vi "实时小时数据单参数上传.vi"() -> (4 "数据发送起始时间":timestamp format="%<%.3X\n%Y/%m/%d>T", 15 "error out":errorcluster)   [LabVIEW 2016, in "数据传输系统.lvlib"]
uses:
  <vilib>/Utility/config.llb/Write Key (String).vi
  <vilib>/Utility/config.llb/NI_LVConfig.lvlib
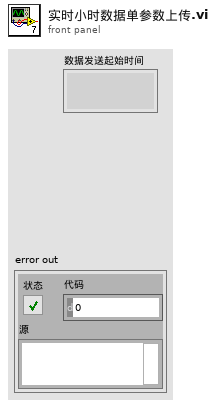
[diagram p1: front panel]
types:
  T1 = cluster{"CODMn":string, "CODCr":string, "DO":string, "铜":string, "PH":string, "氨氮":string, "比电导率":string, "水温":string, "COD":string, "浊度":string, "总氮":string, "总磷":string, "叶绿素a":string, "藻密度":string, "水位":string, "流速":string, "瞬时流量":string, "累积流量":string, "亚硝酸盐":string, "硫化物":string, "ORP":string, "铅":string, "镉":string, "锌":string, "镍":string, "锰":string, "汞":string, "气温":string, "气压":string, "风速":string, "风向":string}
  T2 = cluster{"setini":string, "sysini":string, "hechaini":string, "actualwrite":string, "actualread":string, "datasent":string, "反控命令信息队列":string, "反控与仪器交互":string}
  T3 = cluster{"time1":string, "time2":string, "time3":string, "time4":string, "time5":string, "time6":string, "time7":string, "time8":string, "time9":string, "time10":string, "time11":string, "time12":string, "time13":string, "time14":string, "time15":string, "time16":string, "time17":string, "time18":string, "time19":string, "time20":string, "time21":string, "time22":string, "time23":string, "time24":string, "time25":string, "time26":string, "time27":string, "time28":string, "time29":string, "time30":string, "time31":string}
  T4 = typedef "NI_LVConfig.lvlib/Config Data RefNum.ctl" = refnum<k1>
  T5 = cluster{"水样数据索引[0]":string, "水样数据索引[1]":string, "水样数据索引[2]":string, "水样数据索引[3]":string, "水样数据索引[4]":string, "水样数据索引[5]":string, "水样数据索引[6]":string, "水样数据索引[7]":string, "水样数据索引[8]":string, "水样数据索引[9]":string, "水样数据索引[10]":string, "水样数据索引[11]":string, "水样数据索引[12]":string, "水样数据索引[13]":string, "水样数据索引[14]":string, "水样数据索引[15]":string, "水样数据索引[16]":string, "水样数据索引[17]":string, "水样数据索引[18]":string, "水样数据索引[19]":string, "水样数据索引[20]":string, "水样数据索引[21]":string, "水样数据索引[22]":string, "水样数据索引[23]":string, "水样数据索引[24]":string, "水样数据索引[25]":string, "水样数据索引[26]":string, "水样数据索引[27]":string, "水样数据索引[28]":string, "水样数据索引[29]":string, "水样数据索引[30]":string}
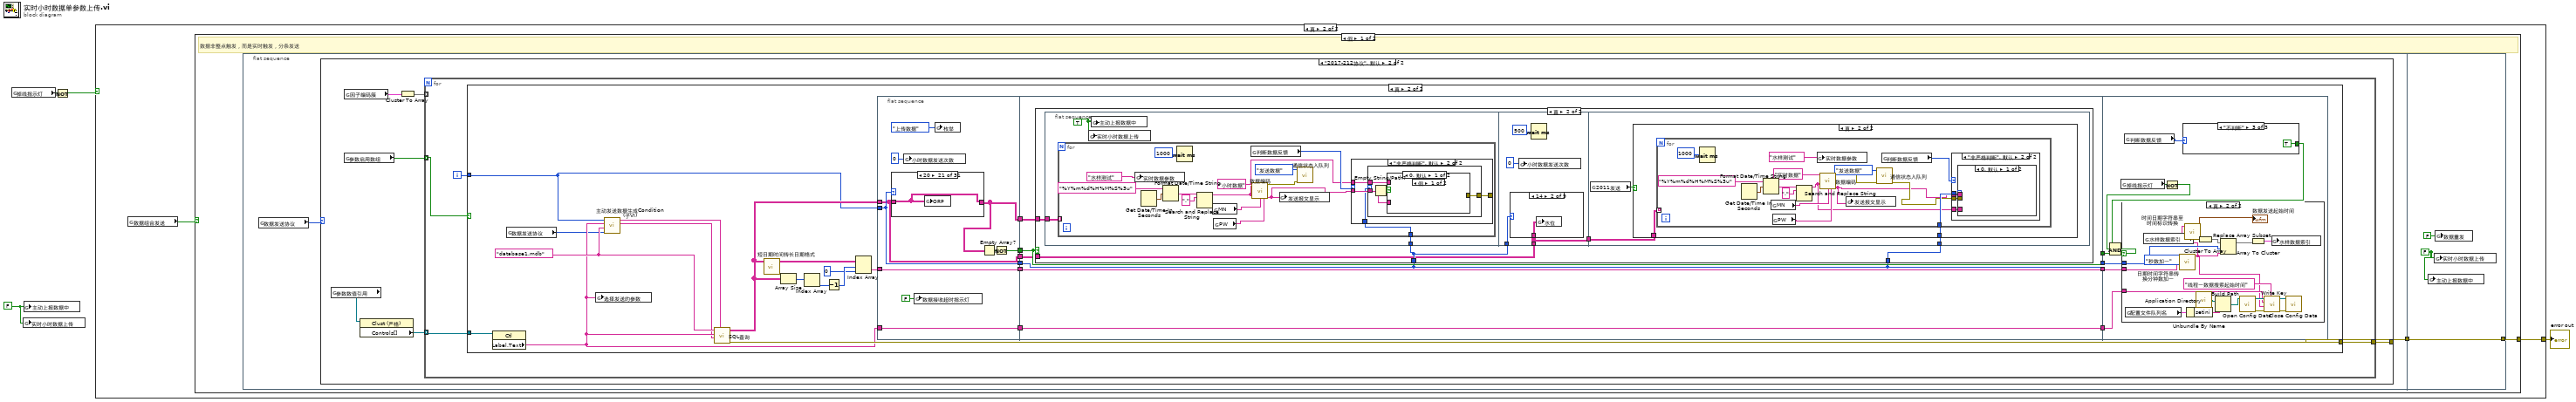
[diagram p0: block diagram]
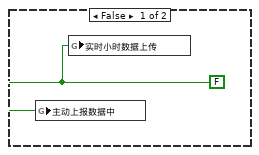
[diagram p2: hidden frame]
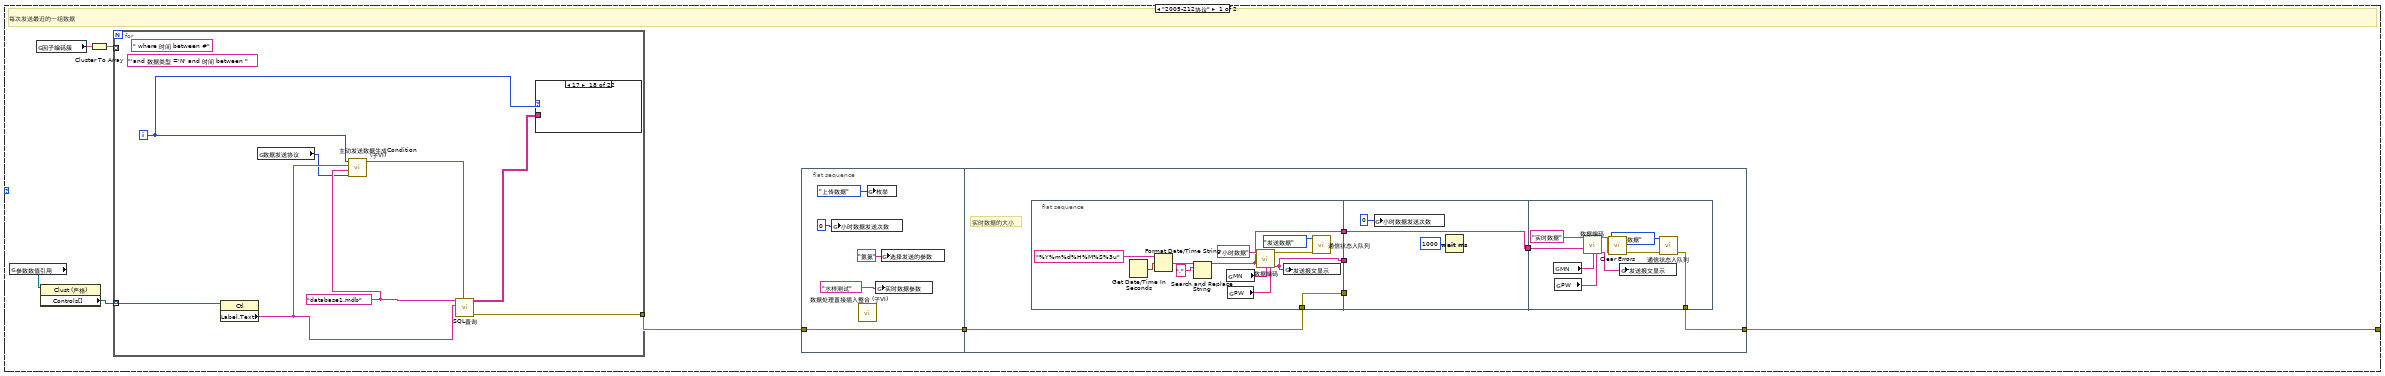
[diagram p3: hidden frame]
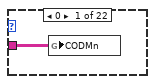
[diagram p4: hidden frame]
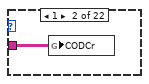
[diagram p5: hidden frame]
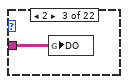
[diagram p6: hidden frame]
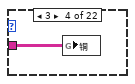
[diagram p7: hidden frame]
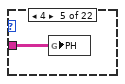
[diagram p8: hidden frame]
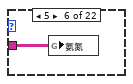
[diagram p9: hidden frame]
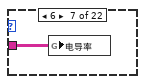
[diagram p10: hidden frame]
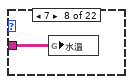
[diagram p11: hidden frame]
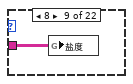
[diagram p12: hidden frame]
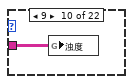
[diagram p13: hidden frame]
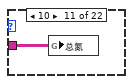
[diagram p14: hidden frame]
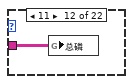
[diagram p15: hidden frame]
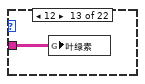
[diagram p16: hidden frame]
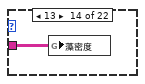
[diagram p17: hidden frame]
diagram:
  w1 = FALSE ("小时数据上传")
  n1 = global read "全局 数据发送重叠.vi" "掉线指示灯"() -> (w4:bool)
  n2 = global write "全局1.vi" "实时小时数据上传"(w1) -> ()
  n3 = global write "全局 数据发送重叠.vi" "主动上报数据中"(w1) -> ()
  n4 = Not(x=w4) -> (.not. x?=w3:bool)
  n5 = case shown="真" w3 {
    tunnel: [_ w7] -> w2
    frame False {
      w5 = FALSE ("小时数据上传")
      n6 = global write "全局 数据发送重叠.vi" "主动上报数据中"(w5) -> ()
      n7 = global write "全局1.vi" "实时小时数据上传"(w5) -> ()
    }
    frame True {
      n8 = global read "断电保存全局.vi" "数据组合发送"() -> (w6:bool)
      n9 = case shown="假" w6 {
        tunnel: [w8 _] -> w7
        frame False {
          # "数据非整点触发，而是实时触发，分条发送"
          n10 = flat-sequence {
            tunnel: [w11] -> w9
            tunnel: [w271] -> w8
            tunnel: w9 -> [w271]
            frame #0 {
              n11 = global read "断电保存全局.vi" "数据发送协议"() -> (w10:enum16{"2005-212协议", "2017-212协议"})
              n12 = case shown="\"2017-212协议\", 默认" w10 {
                tunnel: [w14 w83] -> w11
                frame "2005-212协议" {
                  # "每次发送最近的一组数据"
                  n13 = global read "断电保存全局.vi" "参数数值引用"() -> (w12:refnum<vi>)
                  n14 = global read "断电保存全局.vi" "因子编码簇"() -> (w13:T1)
                  n15 = property class="Clust (严格)"(reference=w12) -> ("Controls[]"=w15:refnum<vi>[])  [unwired: 1 in, 2 out]
                  n16 = Cluster To Array(cluster=w13) -> (array=w18:string[])
                  n17 = for {
                    tunnel: w18 -> [_] mode=indexing
                    tunnel: [w61] -> w17
                    tunnel: w15 -> [w56] mode=indexing
                    i -> [w54]
                    (unwired) " where 时间 between #"
                    w59 = "database1.mdb" ("database")
                    (unwired) "'and 数据类型 ='N' and 时间 between "
                    n18 = property class="Ctl"(reference=w56) -> ("Label.Text"=w60:string)  [unwired: 1 in, 2 out]
                    n19 = global read "断电保存全局.vi" "数据发送协议"() -> (w57:enum16{"2005-212协议", "2017-212协议"})
                    n20 = call "主动发送数据生成Condition(子VI).vi"("数据发送协议"=w57, "database"=w59, "Label.Text"=w60, "数值"=w54) -> ("CONDITION"=w58:string)  [unwired: 6 in, 1 out]
                    n21 = call "SQL查询.vi"("condition"=w58, "table输入"=w60, "database"=w59) -> ("error out"=w61:errorcluster, "data"=w55:string[][])  [unwired: 6 in, 1 out]
                    n22 = case shown="17" w54 {
                      tunnel: w55 -> [w62 w63 w64 w65 w66 w67 w68 w69 w70 w71 w72 w73 w74 w75 _ _ _ _ w76 w77 w78 _]
                      frame 0 {
                        n23 = global write "全局 所有参数.vi" "CODMn"(w62) -> ()
                      }
                      frame 1 {
                        n24 = global write "全局 所有参数.vi" "CODCr"(w63) -> ()
                      }
                      frame 2 {
                        n25 = global write "全局 所有参数.vi" "DO"(w64) -> ()
                      }
                      frame 3 {
                        n26 = global write "全局 所有参数.vi" "铜"(w65) -> ()
                      }
                      frame 4 {
                        n27 = global write "全局 所有参数.vi" "PH"(w66) -> ()
                      }
                      frame 5 {
                        n28 = global write "全局 所有参数.vi" "氨氮"(w67) -> ()
                      }
                      frame 6 {
                        n29 = global write "全局 所有参数.vi" "电导率"(w68) -> ()
                      }
                      frame 7 {
                        n30 = global write "全局 所有参数.vi" "水温"(w69) -> ()
                      }
                      frame 8 {
                        n31 = global write "全局 所有参数.vi" "盐度"(w70) -> ()
                      }
                      frame 9 {
                        n32 = global write "全局 所有参数.vi" "浊度"(w71) -> ()
                      }
                      frame 10 {
                        n33 = global write "全局 所有参数.vi" "总氮"(w72) -> ()
                      }
                      frame 11 {
                        n34 = global write "全局 所有参数.vi" "总磷"(w73) -> ()
                      }
                      frame 12 {
                        n35 = global write "全局 所有参数.vi" "叶绿素"(w74) -> ()
                      }
                      frame 13 {
                        n36 = global write "全局 所有参数.vi" "藻密度"(w75) -> ()
                      }
                      frame 14 {
                      }
                      frame 15 {
                      }
                      frame 16 {
                      }
                      frame 17 {
                      }
                      frame 18 {
                        n37 = global write "全局 所有参数.vi" "亚硝酸盐"(w76) -> ()
                      }
                      frame 19 {
                        n38 = global write "全局 所有参数.vi" "硫化物"(w77) -> ()
                      }
                      frame 20 {
                        n39 = global write "全局 所有参数.vi" "ORP"(w78) -> ()
                      }
                      frame 21, Default {
                      }
                    }
                  }
                  n40 = flat-sequence {
                    tunnel: w17 -> [w19]
                    tunnel: [w19] -> w16
                    tunnel: w16 -> [w27]
                    tunnel: [w26] -> w14
                    frame #0 {
                      n41 = global write "全局 小时数据发送次数.vi" "小时数据发送次数"(0 ("小时数据发送次数")) -> ()
                      n42 = call "数据处理直接插入整合 (子VI).vi"() -> ()  [unwired: 12 in]
                      n43 = global write "全局1.vi" "枚举"(enum16{"返回请求应答", "上传数据", "返回执行结果"}."上传数据" ("枚举")) -> ()
                      n44 = global write "全局 实时数据参数.vi" "实时数据参数"("水样测试" ("实时数据参数")) -> ()
                      n45 = global write "全局 水样时间.vi" "选择发送的参数"("氨氮" ("选择发送的参数")) -> ()
                    }
                    frame #1 {
                      # "实时数据的大小"
                      n46 = flat-sequence {
                        tunnel: [w36] -> w29
                        tunnel: [w31] -> w28
                        tunnel: w27 -> [w31]
                        tunnel: [w30] -> w25
                        tunnel: w29 -> [_]
                        tunnel: w28 -> [_]
                        tunnel: w25 -> [w42]
                        tunnel: [w42] -> w24
                        tunnel: [w47] -> w26
                        tunnel: w24 -> [w46]
                        frame #0 {
                          n47 = Get Date/Time In Seconds() -> (seconds since 1Jan1904=w39:timestamp)
                          n48 = Format Date/Time String(time format string (%c)="%Y%m%d%H%M%S%3u" ("时间格式字符串(%c)"), seconds (now)=w39) -> (date/time string=w40:string)  [unwired: 1 in]
                          n49 = Search and Replace String(input string=w40, search string="." ("搜索字符串")) -> (result string=w30:string)  [unwired: 6 in, 3 out]
                          n50 = global read "断电保存全局.vi" "MN"() -> (w34:string)
                          n51 = global read "断电保存全局.vi" "PW"() -> (w33:string)
                          n52 = call "数据编码.vi"("table输入"="小时数据" ("新元素/子数组"), "QN"=w30, "MN"=w34, "PW"=w33) -> ("错误常量"=w32:errorcluster, "通讯包字符串"=w36:string)  [unwired: 10 in]
                          n53 = global write "全局1.vi" "发送报文显示"(w36) -> ()
                          n54 = call "通信状态入队列.vi"("错误输入（无错误）"=w32, "枚举"=enum16{"打开连接", "发送数据", "读取数据", "数据处理", "关闭连接"}."发送数据") -> ()  [unwired: 9 in, 1 out]
                        }
                        frame #1 {
                          n55 = global write "全局 小时数据发送次数.vi" "小时数据发送次数"(0 ("小时数据发送次数")) -> ()
                          n56 = Wait (ms)(milliseconds to wait=u32 1000 ("等待时间（毫秒）")) -> ()  [unwired: 1 out]
                        }
                        frame #2 {
                          n57 = global read "断电保存全局.vi" "MN"() -> (w49:string)
                          n58 = global read "断电保存全局.vi" "PW"() -> (w50:string)
                          n59 = call "数据编码.vi"("table输入"="实时数据" ("新元素/子数组"), "QN"=w46, "MN"=w49, "PW"=w50) -> ("错误常量"=w48:errorcluster, "通讯包字符串"=w52:string)  [unwired: 10 in]
                          n60 = call <vilib>:"Clear Errors.vi"("error in (no error)"=w48) -> ("error out"=w45:errorcluster)  [unwired: 5 in, 1 out]
                          n61 = global write "全局1.vi" "发送报文显示"(w52) -> ()
                          n62 = call "通信状态入队列.vi"("错误输入（无错误）"=w45, "枚举"=enum16{"打开连接", "发送数据", "读取数据", "数据处理", "关闭连接"}."发送数据") -> ("错误输出"=w47:errorcluster)  [unwired: 9 in]
                        }
                      }
                    }
                  }
                }
                frame "2017-212协议", Default {
                  n63 = global read "断电保存全局.vi" "参数数值引用"() -> (w80:refnum<vi>)
                  n64 = global read "断电保存全局.vi" "参数启用数组"() -> (w79:bool[])
                  n65 = global read "断电保存全局.vi" "因子编码簇"() -> (w81:T1)
                  n66 = property class="Clust (严格)"(reference=w80) -> ("Controls[]"=w82:refnum<vi>[])  [unwired: 1 in, 2 out]
                  n67 = Cluster To Array(cluster=w81) -> (array=w84:string[])
                  n68 = for {
                    tunnel: w84 -> [_] mode=indexing
                    tunnel: [w88] -> w83
                    tunnel: w82 -> [w86] mode=indexing
                    tunnel: w79 -> [w85] mode=indexing
                    i -> [w87]
                    n69 = case shown="真" w85 {
                      tunnel: [_ w101] -> w88
                      tunnel: w87 -> [_ w92]
                      tunnel: w86 -> [_ w91]
                      frame False {
                      }
                      frame True {
                        w100 = "database1.mdb" ("database")
                        n70 = property class="Ctl"(reference=w91) -> ("Label.Text"=w99:string)  [unwired: 1 in, 2 out]
                        n71 = global read "断电保存全局.vi" "数据发送协议"() -> (w98:enum16{"2005-212协议", "2017-212协议"})
                        n72 = global write "全局 水样时间.vi" "选择发送的参数"(w99) -> ()
                        n73 = call "主动发送数据生成Condition(子VI).vi"("数据发送协议"=w98, "database"=w100, "Label.Text"=w99, "数值"=w92) -> ("columns"=w90:string[], "CONDITION"=w104:string)  [unwired: 6 in]
                        n74 = call "SQL查询.vi"("condition"=w104, "columns"=w90, "table输入"=w99, "database"=w100) -> ("error out"=w101:errorcluster, "data"=w95:string[][])  [unwired: 5 in, 1 out]
                        n75 = call "短日期时间转长日期格式.vi"("data"=w95) -> ("输出数组"=w103:string[][])  [unwired: 10 in]
                        n76 = Array Size(array=w95) -> (size(s)=w97:i32[])
                        n77 = Index Array(array=w97) -> (element=w96:i32)  [unwired: 1 in]
                        n78 = Decrement(x=w96) -> (x-1=w94:i32)
                        n79 = Index Array(array=w103, index (row)=w94, index (col)=0 ("禁用的索引 (列)")) -> (element=w102:string)
                        n80 = flat-sequence {
                          tunnel: [w115] -> w113
                          tunnel: [w116] -> w112
                          tunnel: w95 -> [w114]
                          tunnel: w92 -> [w119]
                          tunnel: w99 -> [w121]
                          tunnel: [w121] -> w111
                          tunnel: w102 -> [w120]
                          tunnel: [w120] -> w110
                          tunnel: [w119] -> w109
                          tunnel: [w114] -> w89
                          tunnel: w113 -> [w157]
                          tunnel: w112 -> [w160]
                          tunnel: [w159] -> w108
                          tunnel: w111 -> [w159]
                          tunnel: [w158] -> w107
                          tunnel: w110 -> [w158]
                          tunnel: [w157] -> w106
                          tunnel: [w156] -> w105
                          tunnel: w109 -> [w156]
                          tunnel: w89 -> [w155]
                          tunnel: w108 -> [w245]
                          tunnel: w107 -> [w244]
                          tunnel: w106 -> [w242]
                          tunnel: w105 -> [w243]
                          frame #0 {
                            n81 = case shown="20" w119 {
                              tunnel: w114 -> [w124 w125 w126 w127 w128 w129 w130 w131 w132 w133 w134 w135 w136 w137 _ _ _ _ w142 w143 w144 w145 w146 w147 w148 w149 w150 _ _ _ _]
                              tunnel: [w124 w125 w126 w127 w128 w129 w130 w131 w132 w133 w134 w135 w136 w137 w138 w139 w140 w141 w142 w143 w144 w145 w146 w147 w148 w149 w150 w151 w152 w153 w154] -> w116
                              frame 0, Default {
                                n82 = global write "全局 所有参数.vi" "CODMn"(w124) -> ()
                              }
                              frame 1 {
                                n83 = global write "全局 所有参数.vi" "CODCr"(w125) -> ()
                              }
                              frame 2 {
                                n84 = global write "全局 所有参数.vi" "DO"(w126) -> ()
                              }
                              frame 3 {
                                n85 = global write "全局 所有参数.vi" "铜"(w127) -> ()
                              }
                              frame 4 {
                                n86 = global write "全局 所有参数.vi" "PH"(w128) -> ()
                              }
                              frame 5 {
                                n87 = global write "全局 所有参数.vi" "氨氮"(w129) -> ()
                              }
                              frame 6 {
                                n88 = global write "全局 所有参数.vi" "电导率"(w130) -> ()
                              }
                              frame 7 {
                                n89 = global write "全局 所有参数.vi" "水温"(w131) -> ()
                              }
                              frame 8 {
                                n90 = global write "全局 所有参数.vi" "盐度"(w132) -> ()
                              }
                              frame 9 {
                                n91 = global write "全局 所有参数.vi" "浊度"(w133) -> ()
                              }
                              frame 10 {
                                n92 = global write "全局 所有参数.vi" "总氮"(w134) -> ()
                              }
                              frame 11 {
                                n93 = global write "全局 所有参数.vi" "总磷"(w135) -> ()
                              }
                              frame 12 {
                                n94 = global write "全局 所有参数.vi" "叶绿素"(w136) -> ()
                              }
                              frame 13 {
                                n95 = global write "全局 所有参数.vi" "藻密度"(w137) -> ()
                              }
                              frame 14 {
                                n96 = global read "全局 所有参数.vi" "水位"() -> (w138:string[][])
                              }
                              frame 15 {
                                n97 = global read "全局 所有参数.vi" "流速"() -> (w139:string[][])
                              }
                              frame 16 {
                                n98 = global read "全局 所有参数.vi" "瞬时流量"() -> (w140:string[][])
                              }
                              frame 17 {
                                n99 = global read "全局 所有参数.vi" "累积流量"() -> (w141:string[][])
                              }
                              frame 18 {
                                n100 = global write "全局 所有参数.vi" "亚硝酸盐"(w142) -> ()
                              }
                              frame 19 {
                                n101 = global write "全局 所有参数.vi" "硫化物"(w143) -> ()
                              }
                              frame 20 {
                                n102 = global write "全局 所有参数.vi" "ORP"(w144) -> ()
                              }
                              frame 21 {
                                n103 = global write "全局 所有参数.vi" "铅"(w145) -> ()
                              }
                              frame 22 {
                                n104 = global write "全局 所有参数.vi" "镉"(w146) -> ()
                              }
                              frame 23 {
                                n105 = global write "全局 所有参数.vi" "锌"(w147) -> ()
                              }
                              frame 24 {
                                n106 = global write "全局 所有参数.vi" "镍"(w148) -> ()
                              }
                              frame 25 {
                                n107 = global write "全局 所有参数.vi" "锰"(w149) -> ()
                              }
                              frame 26 {
                                n108 = global write "全局 所有参数.vi" "汞"(w150) -> ()
                              }
                              frame 27 {
                                n109 = global read "全局 所有参数.vi" "气温"() -> (w151:string[][])
                              }
                              frame 28 {
                                n110 = global read "全局 所有参数.vi" "气压"() -> (w152:string[][])
                              }
                              frame 29 {
                                n111 = global read "全局 所有参数.vi" "风速"() -> (w153:string[][])
                              }
                              frame 30 {
                                n112 = global read "全局 所有参数.vi" "风向"() -> (w154:string[][])
                              }
                            }
                            n113 = global write "全局 小时数据发送次数.vi" "小时数据发送次数"(0 ("小时数据发送次数")) -> ()
                            n114 = global write "全局 数据发送重叠.vi" "数据接收超时指示灯"(FALSE ("数据接收超时指示灯")) -> ()
                            n115 = global write "全局1.vi" "枚举"(enum16{"返回请求应答", "上传数据", "返回执行结果"}."上传数据" ("枚举")) -> ()
                            n116 = Empty Array?(array=w116) -> (empty?=w117:bool)
                            n117 = Not(x=w117) -> (.not. x?=w115:bool)
                          }
                          frame #1 {
                            n118 = case shown="真" w157 {
                              tunnel: w160 -> [_ w164]
                              tunnel: w156 -> [_ w163]
                              tunnel: w156 -> [_ w165]
                              tunnel: w155 -> [_ w162]
                              frame False {
                              }
                              frame True {
                                n119 = flat-sequence {
                                tunnel: w163 -> [w168]
                                tunnel: w164 -> [w166]
                                tunnel: w163 -> [w198]
                                tunnel: w162 -> [w197]
                                tunnel: [w197] -> w161
                                tunnel: w165 -> [w209]
                                tunnel: w161 -> [w208]
                                frame #0 {
                                w167 = TRUE ("小时数据上传")
                                n120 = for {
                                tunnel: w168 -> [w183]
                                tunnel: w166 -> [_] mode=indexing
                                n121 = global write "全局 实时数据参数.vi" "实时数据参数"("水样测试" ("实时数据参数")) -> ()
                                n122 = Get Date/Time In Seconds() -> (seconds since 1Jan1904=w180:timestamp)
                                n123 = Format Date/Time String(time format string (%c)="%Y%m%d%H%M%S%3u" ("时间格式字符串(%c)"), seconds (now)=w180) -> (date/time string=w181:string)  [unwired: 1 in]
                                n124 = Wait (ms)(milliseconds to wait=u32 1000 ("等待时间（毫秒）")) -> ()  [unwired: 1 out]
                                n125 = Search and Replace String(input string=w181, search string="." ("搜索字符串")) -> (result string=w170:string)  [unwired: 6 in, 3 out]
                                n126 = global read "断电保存全局.vi" "MN"() -> (w176:string)
                                n127 = global read "断电保存全局.vi" "PW"() -> (w175:string)
                                n128 = global read "断电保存全局.vi" "判断数据反馈"() -> (w172:enum16{"非严格判断", "严格判断", "不判断"})
                                n129 = call "数据编码.vi"("table输入"="小时数据" ("新元素/子数组"), "QN"=w170, "MN"=w176, "PW"=w175) -> ("错误常量"=w173:errorcluster, "通讯包字符串"=w171:string)  [unwired: 10 in]
                                n130 = global write "全局1.vi" "发送报文显示"(w171) -> ()
                                n131 = call "通信状态入队列.vi"("错误输入（无错误）"=w173, "枚举"=enum16{"打开连接", "发送数据", "读取数据", "数据处理", "关闭连接"}."发送数据") -> ()  [unwired: 9 in, 1 out]
                                n132 = case shown="\"非严格判断\", 默认" w172 {
                                tunnel: [_ w187] -> _
                                tunnel: w171 -> [_ w186]
                                tunnel: w183 -> [_ w185]
                                tunnel: w170 -> [_ w184]
                                frame "不判断" {
                                }
                                frame "非严格判断", Default {
                                n133 = case shown="0, 默认" w185 {
                                tunnel: [w190 _] -> w187
                                tunnel: w186 -> [w189 _]
                                tunnel: w184 -> [w188 _]
                                frame 0, Default {
                                n134 = Empty String/Path?(string/path=w189) -> (empty?=w191:bool)
                                n135 = case shown="假" w191 {
                                tunnel: [w195 _] -> w190
                                tunnel: w189 -> [w194 _]
                                tunnel: w188 -> [w192 _]
                                frame False {
                                n136 = global read "断电保存全局.vi" "数据发送通道"() -> (w193:enum16{"TCP", "VISA"})
                                n137 = call "数据补发判定有限循环.vi"("数据输入"=w194, "QN"=w192, "数据发送通道"=w193) -> ("error out"=w195:errorcluster)  [unwired: 8 in]
                                }
                                frame True {
                                }
                                }
                                }
                                frame 14..17, 27..30 {
                                }
                                }
                                }
                                }
                                }
                                n138 = global write "全局1.vi" "实时小时数据上传"(w167) -> ()
                                n139 = global write "全局 数据发送重叠.vi" "主动上报数据中"(w167) -> ()
                                }
                                frame #1 {
                                n140 = case shown="14" w198 {
                                tunnel: w197 -> [_ w200 w201 w202 w203 w204 w205 w206 w207]
                                frame 0, Default {
                                }
                                frame 14 {
                                n141 = global write "全局 所有参数.vi" "水位"(w200) -> ()
                                }
                                frame 15 {
                                n142 = global write "全局 所有参数.vi" "流速"(w201) -> ()
                                }
                                frame 16 {
                                n143 = global write "全局 所有参数.vi" "瞬时流量"(w202) -> ()
                                }
                                frame 17 {
                                n144 = global write "全局 所有参数.vi" "累积流量"(w203) -> ()
                                }
                                frame 27 {
                                n145 = global write "全局 所有参数.vi" "气温"(w204) -> ()
                                }
                                frame 28 {
                                n146 = global write "全局 所有参数.vi" "气压"(w205) -> ()
                                }
                                frame 29 {
                                n147 = global write "全局 所有参数.vi" "风速"(w206) -> ()
                                }
                                frame 30 {
                                n148 = global write "全局 所有参数.vi" "风向"(w207) -> ()
                                }
                                }
                                n149 = global write "全局 小时数据发送次数.vi" "小时数据发送次数"(0 ("小时数据发送次数")) -> ()
                                n150 = Wait (ms)(milliseconds to wait=u32 500 ("等待时间（毫秒）")) -> ()  [unwired: 1 out]
                                }
                                frame #2 {
                                n151 = global read "断电保存全局.vi" "2011发送"() -> (w210:bool)
                                n152 = case shown="真" w210 {
                                tunnel: w209 -> [_ w212]
                                tunnel: w208 -> [_ w211]
                                frame False {
                                }
                                frame True {
                                n153 = for {
                                tunnel: w212 -> [w228]
                                tunnel: w211 -> [_] mode=indexing
                                n154 = Wait (ms)(milliseconds to wait=u32 1000 ("等待时间（毫秒）")) -> ()  [unwired: 1 out]
                                n155 = Get Date/Time In Seconds() -> (seconds since 1Jan1904=w216:timestamp)
                                n156 = Format Date/Time String(time format string (%c)="%Y%m%d%H%M%S%3u" ("时间格式字符串(%c)"), seconds (now)=w216) -> (date/time string=w217:string)  [unwired: 1 in]
                                n157 = global read "断电保存全局.vi" "MN"() -> (w223:string)
                                n158 = global read "断电保存全局.vi" "PW"() -> (w222:string)
                                n159 = Search and Replace String(input string=w217, search string="." ("搜索字符串")) -> (result string=w214:string)  [unwired: 6 in, 3 out]
                                n160 = global write "全局 实时数据参数.vi" "实时数据参数"("水样测试" ("实时数据参数")) -> ()
                                n161 = call "数据编码.vi"("table输入"="实时数据" ("新元素/子数组"), "QN"=w214, "MN"=w223, "PW"=w222) -> ("错误常量"=w224:errorcluster, "通讯包字符串"=w219:string)  [unwired: 10 in]
                                n162 = global write "全局1.vi" "发送报文显示"(w219) -> ()
                                n163 = call "通信状态入队列.vi"("错误输入（无错误）"=w224, "枚举"=enum16{"打开连接", "发送数据", "读取数据", "数据处理", "关闭连接"}."发送数据") -> ("错误输出"=w221:errorcluster)  [unwired: 9 in]
                                n164 = global read "断电保存全局.vi" "判断数据反馈"() -> (w220:enum16{"非严格判断", "严格判断", "不判断"})
                                n165 = case shown="\"非严格判断\", 默认" w220 {
                                tunnel: w219 -> [_ w232]
                                tunnel: w221 -> [_ w231]
                                tunnel: w228 -> [_ w230]
                                tunnel: w214 -> [_ w229]
                                frame "不判断" {
                                }
                                frame "非严格判断", Default {
                                n166 = case shown="0, 默认" w230 {
                                tunnel: w232 -> [w236 _]
                                tunnel: w231 -> [w235 _]
                                tunnel: w229 -> [w233 _]
                                frame 0, Default {
                                n167 = global read "断电保存全局.vi" "数据发送通道"() -> (w234:enum16{"TCP", "VISA"})
                                n168 = call "数据补发判定有限循环.vi"("错误输入（无错误）"=w235, "数据输入"=w236, "QN"=w233, "数据发送通道"=w234) -> ()  [unwired: 7 in, 1 out]
                                }
                                frame 14..17, 27..30 {
                                }
                                }
                                }
                                }
                                }
                                }
                                }
                                }
                                }
                              }
                            }
                          }
                          frame #2 {
                            n169 = global read "全局 数据发送重叠.vi" "掉线指示灯"() -> (w240:bool)
                            n170 = global read "断电保存全局.vi" "判断数据反馈"() -> (w238:enum16{"非严格判断", "严格判断", "不判断"})
                            n171 = Not(x=w240) -> (.not. x?=w239:bool)
                            n172 = case shown="\"不判断\"" w238 {
                              tunnel: [TRUE w247 TRUE] -> w237
                              frame "非严格判断", Default {
                              }
                              frame "严格判断" {
                                n173 = global read "全局 数据发送重叠.vi" "数据接收超时指示灯"() -> (w248:bool)
                                n174 = Not(x=w248) -> (.not. x?=w247:bool)
                              }
                              frame "不判断" {
                              }
                            }
                            n175 = Compound Arithmetic op=AND ("复合运算")(w237, w239, w242) -> (w241:bool)
                            n176 = case shown="真" w241 {
                              tunnel: w244 -> [_ w260]
                              tunnel: w243 -> [_ w254]
                              tunnel: w245 -> [_ w261]
                              frame False {
                              }
                              frame True {
                                n177 = global read "断电保存全局.vi" "配置文件队列名"() -> (w251:T2)
                                n178 = global read "全局 水样时间.vi" "水样数据索引"() -> (w255:T3)
                                n179 = call "日期时间字符串转换分钟数加一.vi"("枚举"=enum16{"分钟数加一", "秒数加一", "小时数加一"}."秒数加一", "data[0]"=w260) -> ("日期/时间字符串"=w253:string)  [unwired: 9 in]
                                n180 = call "时间日期字符串至时间标识转换.vi"("时间日期字符串"=w253) -> ("时间标识"=→"数据发送起始时间":timestamp)  [unwired: 10 in]
                                n181 = Unbundle By Name(w251) -> ("setini"=w250:string)
                                n182 = call <vilib>:"Application Directory.vi"() -> ("Application Directory"=w262:path)
                                n183 = Cluster To Array(cluster=w255) -> (array=w256:string[])
                                n184 = Build Path(base path=w262, name or relative path=w250) -> (appended path=w263:path)
                                n185 = Replace Array Subset(array=w256, new element=w253, index=w254) -> (w257:string[])
                                n186 = call <vilib>:"Open Config Data.vi"("configuration file path"=w263) -> ("error out"=w265:errorcluster, "refnum"=w264:T4)  [unwired: 8 in, 1 out]
                                n187 = Array To Cluster(array=w257) -> (cluster=w258:T5)
                                n188 = call-poly <vilib>:"Write Key.vi"("section"="线程一数据搜索起始时间", "error in (no error)"=w265, "value"=w253, "key"=w261, "refnum"=w264) -> ("error out"=w267:errorcluster, "refnum out"=w266:T4)  [unwired: 4 in, 1 out]
                                n189 = global write "全局 水样时间.vi" "水样数据索引"(w258) -> ()
                                n190 = call <vilib>:"Close Config Data.vi"("error in (no error)"=w267, "refnum"=w266) -> ()  [unwired: 8 in, 2 out]
                              }
                            }
                          }
                        }
                      }
                    }
                  }
                }
              }
            }
            frame #1 {
              w270 = FALSE ("小时数据上传")
              n191 = global write "全局 数据发送重叠.vi" "主动上报数据中"(w270) -> ()
              n192 = global write "全局1.vi" "实时小时数据上传"(w270) -> ()
              n193 = global write "断电保存全局.vi" "数据重发"(FALSE ("数据重发")) -> ()
            }
          }
        }
        frame True {
          # "数据整点触发，整条发送"
          n194 = flat-sequence {
            frame #0 {
              n195 = global read "断电保存全局.vi" "数据发送通道"() -> (w272:enum16{"TCP", "VISA"})
              n196 = global read "断电保存全局.vi" "MN"() -> (w274:string)
              n197 = global read "断电保存全局.vi" "PW"() -> (w273:string)
              n198 = call "数据全参数一起发送整点触发.vi"("数据发送通道"=w272, "PW"=w273, "MN"=w274) -> ()  [unwired: 8 in]
            }
            frame #1 {
              w275 = FALSE ("主动上报数据中")
              n199 = global write "全局 数据发送重叠.vi" "主动上报数据中"(w275) -> ()
              n200 = global write "全局1.vi" "实时小时数据上传"(w275) -> ()
            }
          }
        }
      }
    }
  }
  "error out" <- w2
